vi "Check Data Plugin.vi"(0 "reference in":refnum<class "HeadAcousticHDF.lvclass">, 5 "error in (no error)":errorcluster) -> (13 "HDF Plugin OK?":bool, 14 "reference out":refnum<class "HeadAcousticHDF.lvclass">, 19 "error out":errorcluster)   [LabVIEW 2022 SP3, in "HeadAcousticHDF.lvclass"]
uses:
  HeadAcousticHDF.lvclass
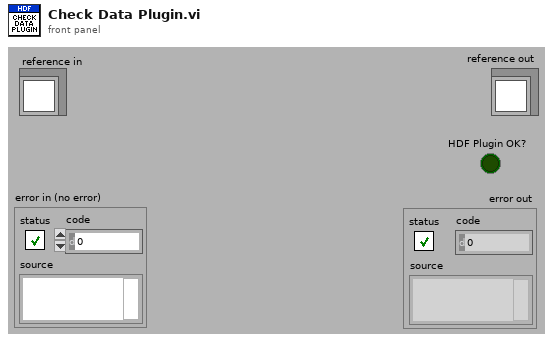
[diagram p1: front panel]
types:
  T1 = typedef "HeadAcousticHDF.lvclass/ObjectAttributes.ctl" = cluster{"Time Data":refnum<class "GSwFormDSP.lvclass">, "Data Plugin Name":string, "Additional Data Plugin Name":string, "New Time Data Obj?":bool}
  T2 = typedef "usiPluginInformation.ctl" = cluster{"name":string, "version":string, "type":string, "read-only?":bool, "extensions":string[]}
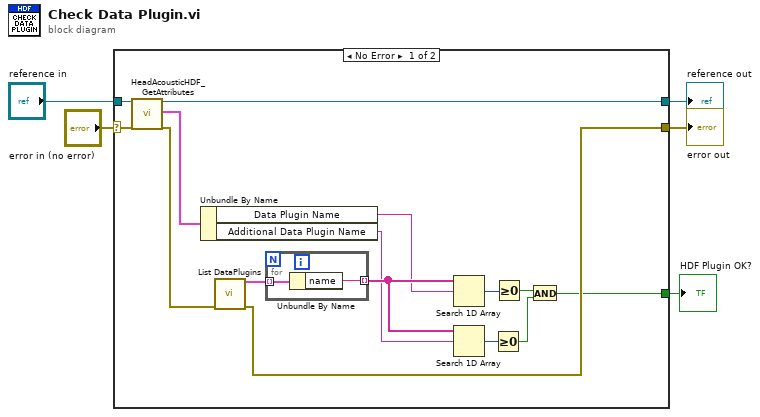
[diagram p0: block diagram]
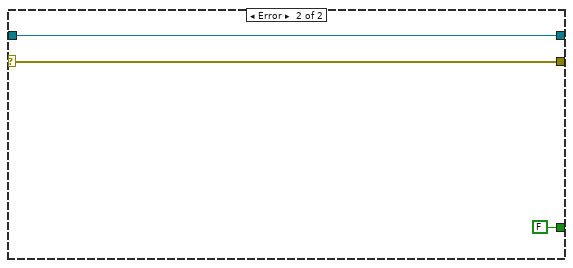
[diagram p2: hidden frame]
diagram:
  n1 = case shown="No Error" "error in (no error)" {
    selector: "error in (no error)" -> [w20 w25]
    tunnel: [w11 w25] -> w4
    tunnel: [w19 w24] -> w2
    tunnel: "reference in" -> [w18 w24]
    tunnel: [w6 FALSE] -> w1
    frame No Error {
      n2 = call "HeadAcousticHDF_GetAttributes.vi"("reference in"=w18, "error in (no error)"=w20) -> ("reference out"=w19:refnum<class "HeadAcousticHDF.lvclass">, "attributes"=w17:T1, "error out"=w16:errorcluster)  [unwired: 14 in, 1 out]
      n3 = Unbundle By Name(w17) -> ("Data Plugin Name"=w13:string, "Additional Data Plugin Name"=w12:string)
      n4 = call <vilib>:"List DataPlugins.vi"("error in (no error)"=w16) -> ("DataPlugin information"=w15:T2[], "error out"=w11:errorcluster)  [unwired: 13 in]
      n5 = for {
        tunnel: w15 -> [w22] mode=indexing
        tunnel: [w21] -> w14 mode=indexing
        n6 = Unbundle By Name(w22) -> ("name"=w21:string)
      }
      n7 = Search 1D Array(1D array=w14, element=w13) -> (index of element=w10:i32)  [unwired: 1 in]
      n8 = Search 1D Array(1D array=w14, element=w12) -> (index of element=w9:i32)  [unwired: 1 in]
      n9 = Greater Or Equal To 0?(x=w9) -> (x >= 0?=w7:bool)
      n10 = Greater Or Equal To 0?(x=w10) -> (x >= 0?=w8:bool)
      n11 = And(x=w8, y=w7) -> (x .and. y?=w6:bool)
    }
    frame Error {
    }
  }
  "error out" <- w4
  "reference out" <- w2
  "HDF Plugin OK?" <- w1
